vi "RTUStringToASCString.vi"(8 "RTUString":string) -> (0 "ASCString":string)   [LabVIEW 2023]
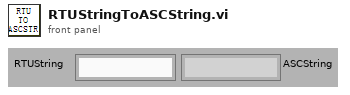
[diagram p1: front panel]
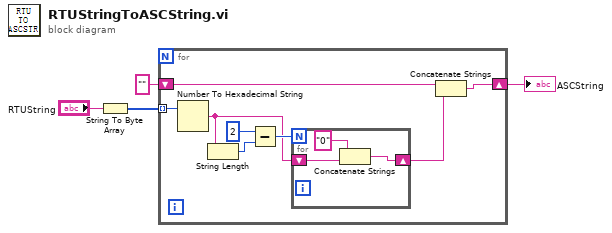
[diagram p0: block diagram]
diagram:
  n1 = String To Byte Array(string="RTUString") -> (unsigned byte array=w3:u8[])
  n2 = for {
    tunnel: w3 -> [w12] mode=indexing
    shift-right: [w10] -> w1
    shift-left: "" -> [w11]
    n3 = Number To Hexadecimal String(2:w12) -> (0:w6:string)  [unwired: 1 in]
    n4 = String Length(string=w6) -> (length=w8:i32)
    n5 = Subtract(x=2, y=w8) -> (x-y=w7:i32)
    n6 = for {
      N: w7 -> [_]
      shift-right: [w13] -> w5
      shift-left: w6 -> [w14]
      n7 = Concatenate Strings("0", w14) -> (w13:string)
    }
    n8 = Concatenate Strings(w11, w5) -> (w10:string)
  }
  "ASCString" <- w1
